vi "PMBus Write Byte Ext.vi"(1 "PEC":u8, 4 "Data":u8, 5 "CommandCode":u8, 6 "CommandCodeExt":u8, 7 "SlaveAddr":u8, 9 "PMBusIndex":i32, 10 "DevIndex":i32, 11 "DevType":i32) -> (3 "function return":i32)   [LabVIEW 2010, in "ControlPMBus.lvlib"]
doc: "int WINAPI PMBus_WriteByteExt(int DevType,int DevIndex,int PMBusIndex,unsigned char SlaveAddr,unsigned char CommandCodeExt,unsigned char CommandCode,unsigned char Data,unsigned char PEC);"
uses:
  ControlPMBus.lvlib
  ControlPMBus/Ginkgo_Driver.dll
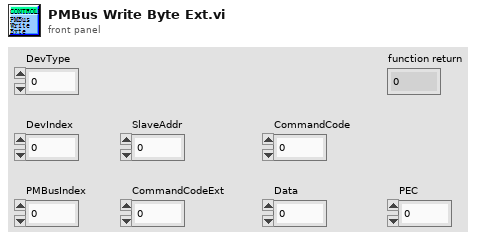
[diagram p1: front panel]
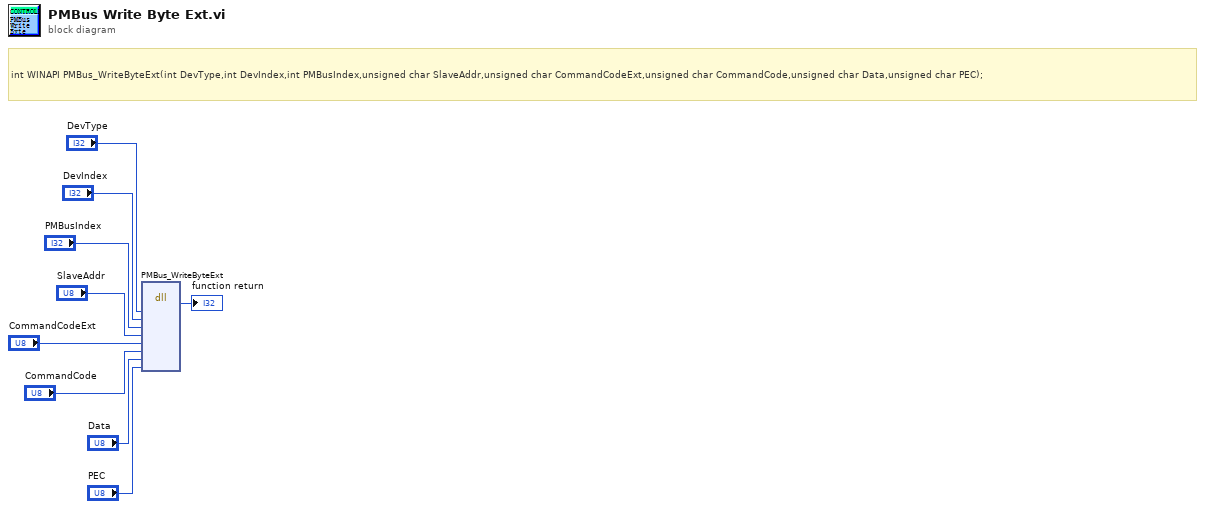
[diagram p0: block diagram]
diagram:
  # "int WINAPI PMBus_WriteByteExt(int DevType,int DevIndex,int PMBusIndex,unsigned char SlaveAddr,unsigned char CommandCodeExt,unsigned char CommandCode,unsigned char Data,unsigned char PEC);"
  n1 = dll-call lib="E:/Project/vt_ginkgo/truck/Ginkgo Driver/vs2010/Ginkgo_USB-I2C&SPI&CAN_API_v2.0.3.3/lib/labview_32bit/ControlPMBus/Ginkgo_Driver.*" fn="PMBus_WriteByteExt"("DevType"="DevType", "DevIndex"="DevIndex", "PMBusIndex"="PMBusIndex", "SlaveAddr"="SlaveAddr", "CommandCodeExt"="CommandCodeExt", "CommandCode"="CommandCode", "Data"="Data", "PEC"="PEC") -> (→"function return":i32)  [unwired: 11 in, 2 out]
